vi "LabFrog.vi"(8 "Simutation":bool, 11 "FROG path":path=path "C:/FROG") -> (0 "error out":errorcluster, 3 "FROG data":T1[](array[typedef])=[{"Delay increment"=36.8, "Center Wavelength"=809.3, "Frog Error was"=0.0344, "Temporal FWHM"=100.0, "Spectral FWHM"=7.96, "FWHM Time-Bandwidth Product"=0.364, "RMS Time-Bandwidth Product"=0.85}, {"Delay increment"=36.8, "Center Wavelength"=809.3, "Frog Error was"=0.036, "Temporal FWHM"=98.9, "Spectral FWHM"=9.04, "FWHM Time-Bandwidth Product"=0.408, "RMS Time-Bandwidth Product"=0.858}])   [LabVIEW 2014]
doc: "LabFROG \n\nExtract data value from FROG file\n\nAndré Romero - 2022\nandretec@ifsc.usp.br"
uses:
  FROG.ctl
  <vilib>/regexp/Match Regular Expression.xnode
panel:
  out "index":i32=13
  out "max value (ms)":u32=2
  out "Delay":u32[](array[numeric])=[0, 1, 1, 0, 1, 1, 1, 1, 0, 1, 0, 1, 0, 2, 0, 1, 0, 1, 1, 0, 1, 1, 0, 2, 1, 1, 1, 1, 1, 0, 1, 0, 1, 1, 1, 0, 1, 0, 1]
  out "FROG data":string[][](array[string])=[["32", "32"], ["36.8", "36.8"], ["809.3", "809.3"], ["0.0344", "0.036"], ["100", "98.9"], ["7.96", "9.04"], ["0.364", "0.408"], ["0.85", "0.858"], ["", ""]]
  out "FROG text data":string="Grid characteristics were: 32 points; Delay increment: 36.8 fs; Center Wavelength: 809.3 nm\nFrog Error was: 0.036\nTemporal FWHM: 98.9 fs\nSpectral FWHM: 9.04 nm\nFWHM Time-Bandwidth Product: 0.408\nRMS Time-Bandwidth Product: 0.858\n"
  out "filenames":string[](array[string])=["2022-05-26_10-35-10_ESpectral.dat", "2022-05-26_10-35-10_ETemporal.dat", "2022-05-26_10-35-10_ExpFrog.bmp", "2022-05-26_10-35-10_ExpFrog.dat", "2022-05-26_10-35-10_ExpFrog.jpg", "2022-05-26_10-35-10_Frog.dat", "2022-05-26_10-35-10_RawData.bmp", "2022-05-26_10-35-10_RawData.dat", "2022-05-26_10-35-10_RawData.jpg", "2022-05-26_10-35-10_RawData.png", "2022-05-26_10-35-10_RetrFrog.bmp", "2022-05-26_10-35-10_RetrFrog.dat", "2022-05-26_10-35-10_RetrFrog.jpg", "2022-05-26_10-35-10_screenShot.bmp", "2022-05-26_10-35-10_ss-colorpanel.jpg", "2022-05-26_10-35-10_ss-exper.jpg", "2022-05-26_10-35-10_ss-retrieved.jpg", "2022-05-26_10-35-10_ss-spectral.jpg", "2022-05-26_10-35-10_ss-temporal.jpg", "2022-05-26_10-35-16_ESpectral.dat", "2022-05-26_10-35-16_ETemporal.dat", "2022-05-26_10-35-16_ExpFrog.bmp", "2022-05-26_10-35-16_ExpFrog.dat", "2022-05-26_10-35-16_ExpFrog.jpg", "2022-05-26_10-35-16_Frog.dat", "2022-05-26_10-35-16_RawData.bmp", "2022-05-26_10-35-16_RawData.dat", "2022-05-26_10-35-16_RawData.jpg", "2022-05-26_10-35-16_RawData.png", "2022-05-26_10-35-16_RetrFrog.bmp", "2022-05-26_10-35-16_RetrFrog.dat", "2022-05-26_10-35-16_RetrFrog.jpg", "2022-05-26_10-35-16_screenShot.bmp", "2022-05-26_10-35-16_ss-colorpanel.jpg", "2022-05-26_10-35-16_ss-exper.jpg", "2022-05-26_10-35-16_ss-retrieved.jpg", "2022-05-26_10-35-16_ss-spectral.jpg", "2022-05-26_10-35-16_ss-temporal.jpg", "Thumbs.db"]
  # "[1] Delay increment"
  # "[2] Center Wavelength"
  # "[3] Frog Error was"
  # "[4] Temporal FWHM"
  # "[5] Spectral FWHM"
  # "[6] FWHM Time-Bandwidth Product"
  # "[7] RMS Time-Bandwidth Product"
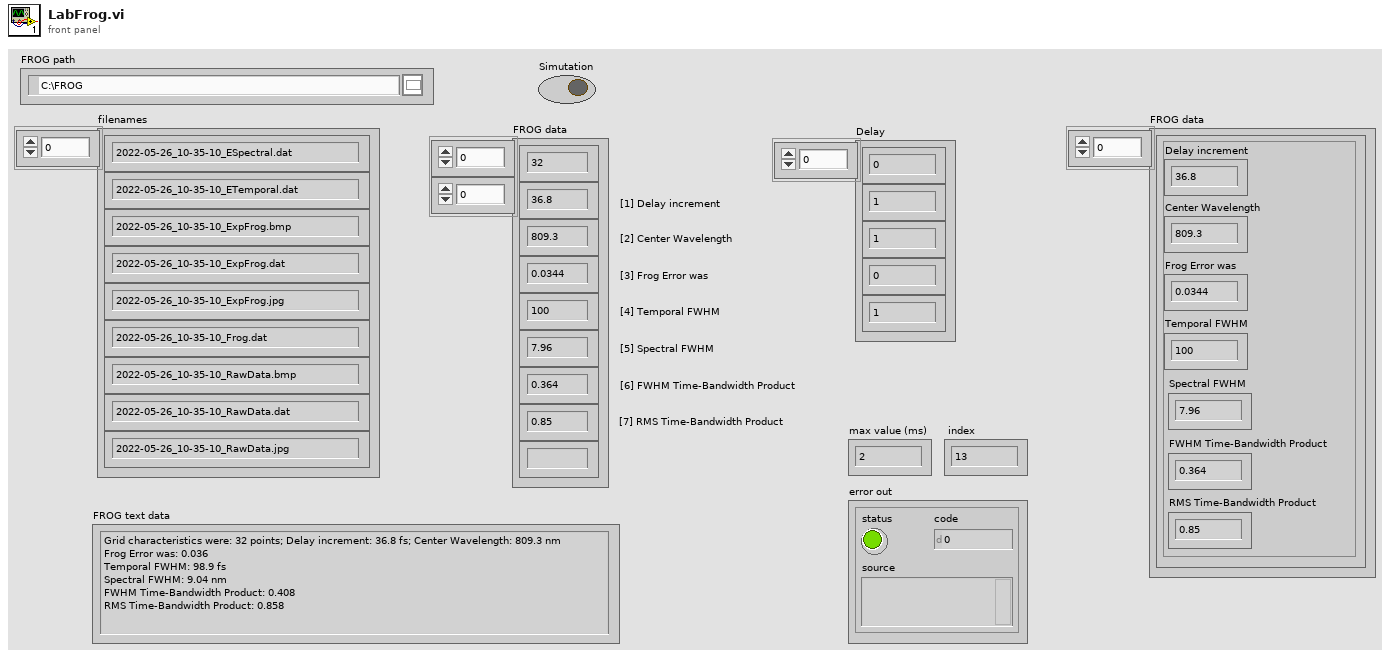
[diagram p1: front panel]
types:
  T1 = typedef "FROG.ctl" = cluster{"Delay increment":dbl, "Center Wavelength":dbl, "Frog Error was":dbl, "Temporal FWHM":dbl, "Spectral FWHM":dbl, "FWHM Time-Bandwidth Product":dbl, "RMS Time-Bandwidth Product":dbl}
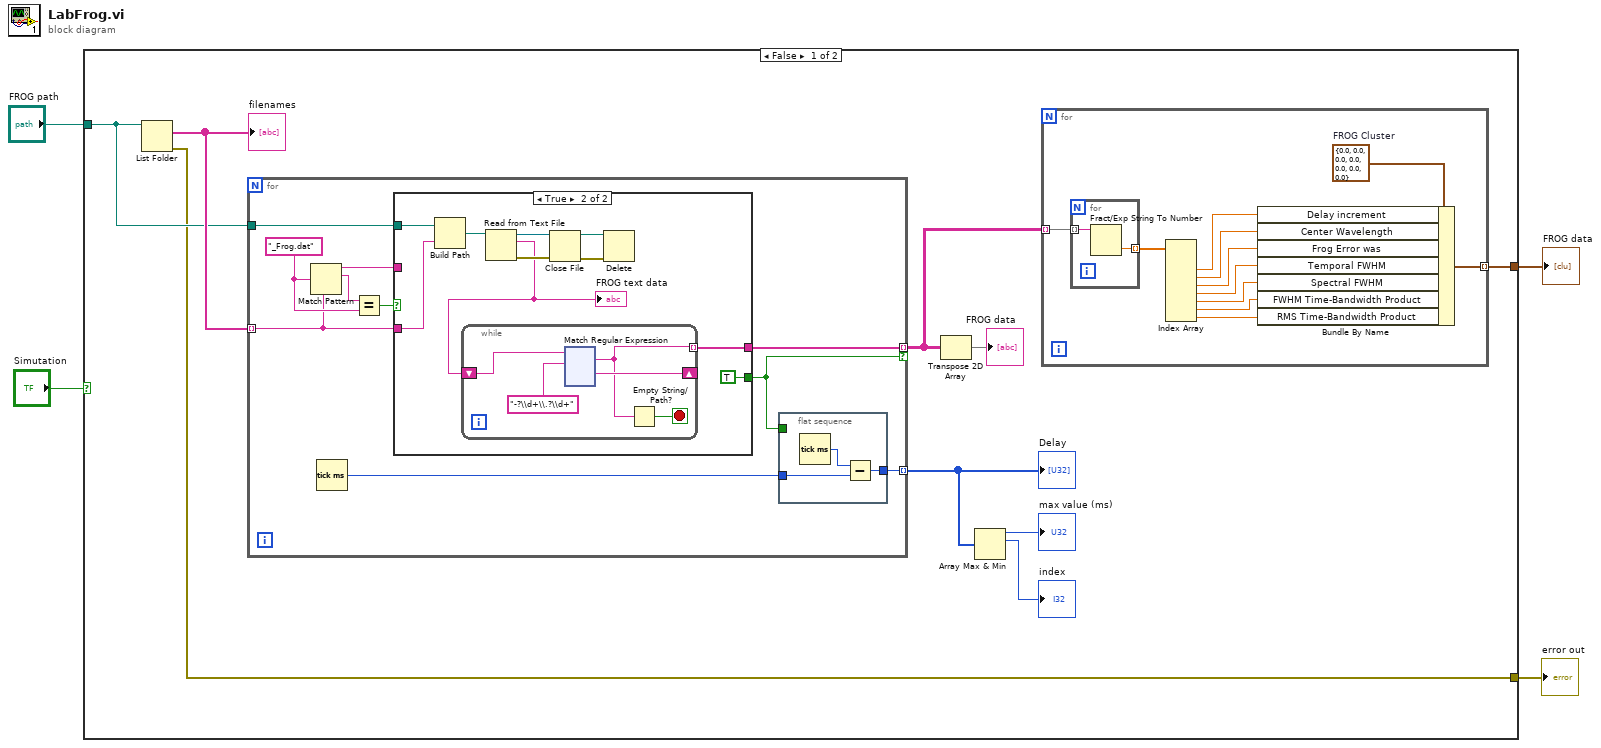
[diagram p0: block diagram]
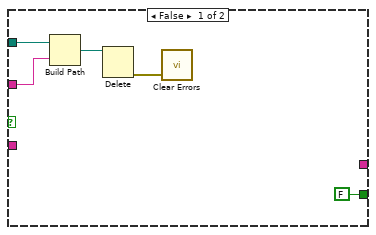
[diagram p2: hidden frame]
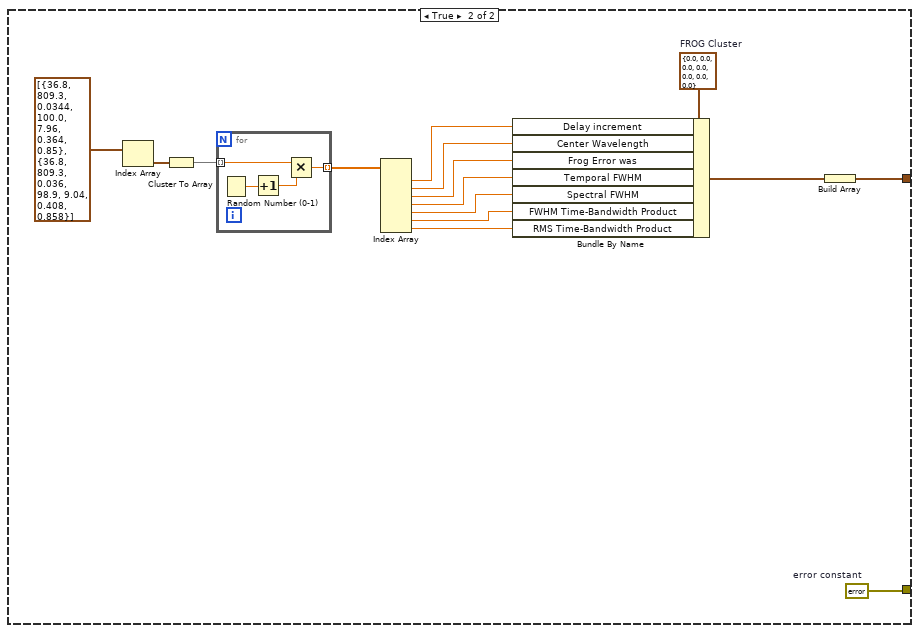
[diagram p3: hidden frame]
diagram:
  n1 = case shown="False" "Simutation" {
    tunnel: "FROG path" -> [w12 _]
    tunnel: [w6 w177] -> w3
    tunnel: [w5 w188] -> w2
    frame False {
      n2 = List Folder(path=w12) -> (filenames=w13:string[], error out=w5:errorcluster)  [unwired: 3 in, 2 out]
      "filenames" <- w13
      n3 = for {
        tunnel: w13 -> [w33] mode=indexing
        tunnel: w12 -> [w32]
        tunnel: [w27] -> w7 mode=indexing if=w30
        tunnel: [w28] -> w10 mode=indexing
        w35 = "_Frog.dat" ("regular expression")
        n4 = Match Pattern(string=w33, regular expression=w35) -> (before substring=w31:string, match substring=w36:string)  [unwired: 1 in, 2 out]
        n5 = Tick Count (ms)() -> (millisecond timer value=w29:u32)
        n6 = Equal?(x=w36, y=w35) -> (x = y?=w34:bool)
        n7 = case shown="True" w34 {
          tunnel: w33 -> [_ w53]
          tunnel: w32 -> [w43 w54]
          tunnel: [_ w51] -> w27
          tunnel: [FALSE TRUE] -> w30
          tunnel: w31 -> [w42 _]
          frame False {
            n8 = Build Path(base path=w43, name or relative path=w42) -> (appended path=w41:path)
            n9 = Delete(path (use dialog)=w41) -> (error out=w40:errorcluster)  [unwired: 4 in, 2 out]
            n10 = call <vilib>:"Clear Errors.vi"("error in (no error)"=w40) -> ()  [unwired: 5 in, 2 out]
          }
          frame True {
            n11 = Build Path(base path=w54, name or relative path=w53) -> (appended path=w52:path)
            n12 = Read from Text File(file (use dialog)=w52) -> (refnum out=w50:refnum<file>, text=w48:string, error out=w49:errorcluster)  [unwired: 3 in, 1 out]
            "FROG text data" <- w48
            n13 = while {
              shift-right: [w57] -> _
              shift-left: w48 -> [w59]
              tunnel: [w56] -> w51 mode=indexing
              stop <- w55 stop-if-true
              n14 = xnode "Match Regular Expression"("input string"=w59, "regular expression"="-?\\d+\\.?\\d+") -> ("whole match"=w56:string, "after match"=w57:string)  [unwired: 4 in, 3 out]
              n15 = Empty String/Path?(string/path=w56) -> (empty?=w55:bool)
            }
            n16 = Close File(refnum=w50, error in=w49) -> (path=w45:path, error out=w46:errorcluster)
            n17 = Delete(path (use dialog)=w45, error in=w46) -> ()  [unwired: 3 in, 3 out]
          }
        }
        n18 = flat-sequence {
          tunnel: w30 -> [_]
          tunnel: w29 -> [w38]
          tunnel: [w37] -> w28
          frame #0 {
            n19 = Tick Count (ms)() -> (millisecond timer value=w39:u32)
            n20 = Subtract(x=w39, y=w38) -> (x-y=w37:u32)
          }
        }
      }
      "Delay" <- w10
      n21 = Transpose 2D Array(2D array=w7) -> (transposed array=→"FROG data":string[][])
      n22 = Array Max & Min(array=w10) -> (max value=→"max value (ms)":u32, max index (indices)=→"index":i32)  [unwired: 2 out]
      n23 = for {
        tunnel: w7 -> [w24] mode=indexing
        tunnel: [w14] -> w6 mode=indexing
        w22 = T1 {"Delay increment"=0.0, "Center Wavelength"=0.0, "Frog Error was"=0.0, "Temporal FWHM"=0.0, "Spectral FWHM"=0.0, "FWHM Time-Bandwidth Product"=0.0, "RMS Time-Bandwidth Product"=0.0}  # FROG Cluster
        n24 = for {
          tunnel: w24 -> [w26] mode=indexing
          tunnel: [w25] -> w23 mode=indexing
          n25 = Fract/Exp String To Number(string=w26) -> (number=w25:dbl)  [unwired: 3 in, 1 out]
        }
        n26 = Index Array(array=w23) -> (element #2=w15:dbl, element #3=w16:dbl, element #4=w17:dbl, element #5=w18:dbl, element #6=w19:dbl, element #7=w20:dbl, element #8=w21:dbl)  [unwired: 8 in, 1 out]
        n27 = Bundle By Name(cluster=w22, "Delay increment"=w15, "Center Wavelength"=w16, "Frog Error was"=w17, "Temporal FWHM"=w18, "Spectral FWHM"=w19, "FWHM Time-Bandwidth Product"=w20, "RMS Time-Bandwidth Product"=w21) -> (w14:T1)
      }
    }
    frame True {
      w184 = T1 {"Delay increment"=0.0, "Center Wavelength"=0.0, "Frog Error was"=0.0, "Temporal FWHM"=0.0, "Spectral FWHM"=0.0, "FWHM Time-Bandwidth Product"=0.0, "RMS Time-Bandwidth Product"=0.0}  # FROG Cluster
      w188 = errorcluster {"status"=FALSE, "code"=0, "source"=""}  # error constant
      n28 = Index Array(array=T1[] [{"Delay increment"=36.8, "Center Wavelength"=809.3, "Frog Error was"=0.0344, "Temporal FWHM"=100.0, "Spectral FWHM"=7.96, "FWHM Time-Bandwidth Product"=0.364, "RMS Time-Bandwidth Product"=0.85}, {"Delay increment"=36.8, "Center Wavelength"=809.3, "Frog Error was"=0.036, "Temporal FWHM"=98.9, "Spectral FWHM"=9.04, "FWHM Time-Bandwidth Product"=0.408, "RMS Time-Bandwidth Product"=0.858}] ("FROG data")) -> (element=w187:T1)  [unwired: 1 in]
      n29 = Cluster To Array(cluster=w187) -> (array=w186:dbl[])
      n30 = for {
        tunnel: w186 -> [w192] mode=indexing
        tunnel: [w190] -> w183 mode=indexing
        n31 = Random Number (0-1)() -> (number: 0 to 1=w191:dbl)
        n32 = Increment(x=w191) -> (x+1=w189:dbl)
        n33 = Multiply(x=w192, y=w189) -> (x*y=w190:dbl)
      }
      n34 = Index Array(array=w183) -> (element #1=w182:dbl, element #2=w181:dbl, element #3=w180:dbl, element #4=w179:dbl, element #5=w178:dbl, element #6=w175:dbl, element #7=w174:dbl)  [unwired: 7 in]
      n35 = Bundle By Name(cluster=w184, "Delay increment"=w182, "Center Wavelength"=w181, "Frog Error was"=w180, "Temporal FWHM"=w179, "Spectral FWHM"=w178, "FWHM Time-Bandwidth Product"=w175, "RMS Time-Bandwidth Product"=w174) -> (w176:T1)
      n36 = Build Array(w176) -> (w177:T1[])
    }
  }
  "FROG data" <- w3
  "error out" <- w2
